vi "Add Tag Token.vi"(8 "Error In":errorcluster, 11 "Parser In":refnum<class "Parser.lvclass">) -> (0 "Error Out":errorcluster, 3 "Parser Out":refnum<class "Parser.lvclass">)   [LabVIEW 2017, in "Mustache.lvlib" / "Parser.lvclass"]
uses:
  Parser.lvclass
  Parser.lvclass/Parser.ctl
  Tokens/Public/Tag/Public/Controls/Types.ctl
  Tokens/Public/Tag/Tag.lvclass
  D:/Users/cfield/Code/Field R&D Services/Mustache/feature-lv-original-parser/src/Mustache/Public/Tokens/Public/Abstract/Abstract.lvclass
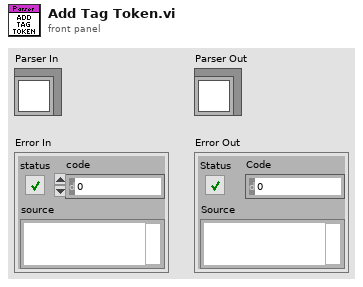
[diagram p1: front panel]
types:
  T1 = typedef "Mustache.lvlib/Tokens.lvlib/Tag.lvclass/Types.ctl" = enum16{"HTML Escaped Variable", "HTML Unescaped Variable", "Unescaped Variable", "Begin Section", "Invert Section", "End Section", "Comment", "Partial", "Set Delimiter"}
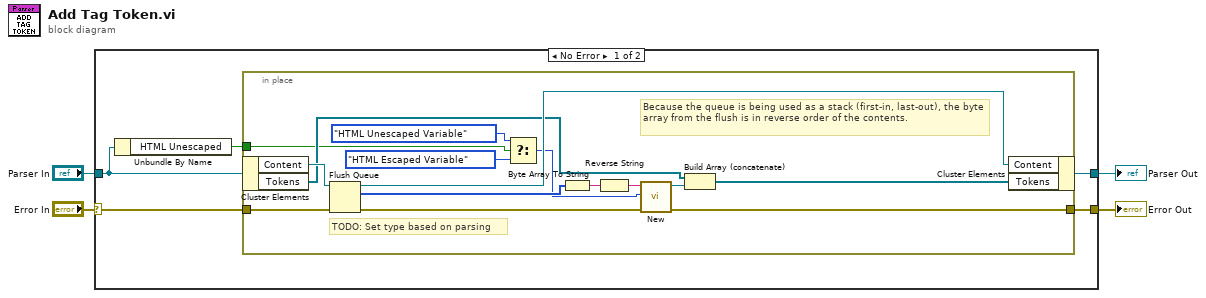
[diagram p0: block diagram]
diagram:
  n1 = case shown="No Error" "Error In" {
    selector: "Error In" -> [w7 w25]
    tunnel: [w9 w25] -> w4
    tunnel: [w8 w26] -> w3
    tunnel: "Parser In" -> [w6 w26]
    frame No Error {
      n2 = Unbundle By Name(w6) -> ("HTML Unescaped"=w5:bool)
      n3 = in-place {
        in-place-border: [w20] -> w9
        in-place-border: w7 -> [w16]
        in-place-border: w5 -> [w13]
        # "TODO: Set type based on parsing"
        # "Because the queue is being used as a stack (first-in, last-out), the byte array from the flush is in reverse order of the contents."
        n4 = in-place-cluster #1(w6) -> ("Content"=w24:refnum<queue>, "Tokens"=w19:refnum<class "Abstract.lvclass">[])
        n5 = Flush Queue(queue=w24, error in (no error)=w16) -> (queue out=w23:refnum<queue>, remaining elements=w22:u8[], error out=w21:errorcluster)
        n6 = Select(t=Types."HTML Unescaped Variable", s=w13, f=Types."HTML Escaped Variable" ("Type")) -> (s? t:f=w11:T1)
        n7 = Byte Array To String(unsigned byte array=w22) -> (string=w15:string)
        n8 = Reverse String(1:w15) -> (0:w14:string)
        n9 = call "New.vi"("Error In"=w21, "Type"=w11, "Key"=w14) -> ("Error Out"=w20:errorcluster, "Tag"=w18:refnum<class "Tag.lvclass">)  [unwired: 7 in]
        n10 = Build Array (concatenate)(w19, w18) -> (w17:refnum<class "Abstract.lvclass">[])
        n11 = in-place-cluster #1("Content"=w23, "Tokens"=w17) -> (w8:refnum<class "Parser.lvclass">)
      }
    }
    frame Error {
    }
  }
  "Error Out" <- w4
  "Parser Out" <- w3
